vi "Request Data JSON.vi"(8 "error in (no error)":errorcluster, 11 "GetSceneItemEnabled in":refnum<class "GetSceneItemEnabled.lvclass">) -> (0 "error out":errorcluster, 2 "Request Data JSON":string, 3 "GetSceneItemEnabled out":refnum<class "GetSceneItemEnabled.lvclass">)   [LabVIEW 2020, in "obs-websocket.lvlib" / "GetSceneItemEnabled.lvclass"]
uses:
  GetSceneItemEnabled.lvclass
  GetSceneItemEnabled.lvclass/GetSceneItemEnabled.ctl
  8b3391d9-ccc5-48a8-9ab5-f487bbe7d852.vi
  <vilib>/JDP Science/JSONtext/Variant to JSON Text.vi
  <vilib>/JDP Science/JSONtext/LVClass Serializer/JSONtext LVClass Serializer.lvclass
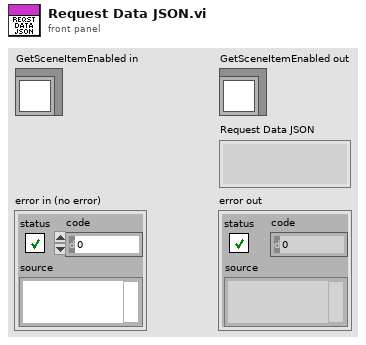
[diagram p1: front panel]
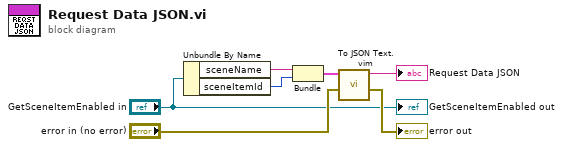
[diagram p0: block diagram]
diagram:
  n1 = Unbundle By Name("GetSceneItemEnabled in") -> ("sceneName"=w4:string, "sceneItemId"=w3:i32)
  n2 = Bundle("sceneName"=w4, "sceneItemId"=w3) -> (w2:cluster{"sceneName":string, "sceneItemId":i32})  [unwired: 1 in]
  n3 = call "To JSON Text.vim"("error in (no error)"="error in (no error)", "Anything"=w2) -> ("error out"=→"error out":errorcluster, "<JSON>"=→"Request Data JSON":string)  [unwired: 8 in]
  "GetSceneItemEnabled out" <- "GetSceneItemEnabled in"
